vi "MCLB Populate.vi"(6 "Item Names[][]":string[][](array[string]), 8 "error in (no error)":errorcluster, 9 "Column Header Strings[]":string[](array[string]), 10 "Row Header Strings[]":string[](array[string]), 11 "View in":refnum<class "MCListbox View.lvclass">) -> (0 "error out":errorcluster, 3 "View out":refnum<class "MCListbox View.lvclass">)   [LabVIEW 2013, in "SET Project Editor.lvlib" / "MCListbox View.lvclass"]
uses:
  MCListbox View.lvclass
  MCListbox View.lvclass/MCListbox View.ctl
  SET Project Editor.lvlib
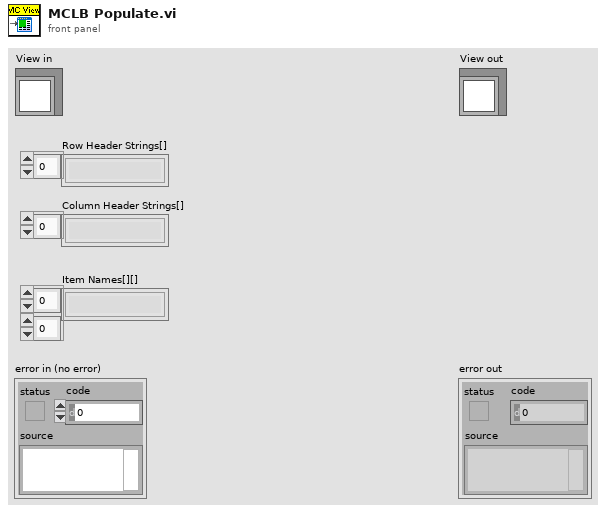
[diagram p1: front panel]
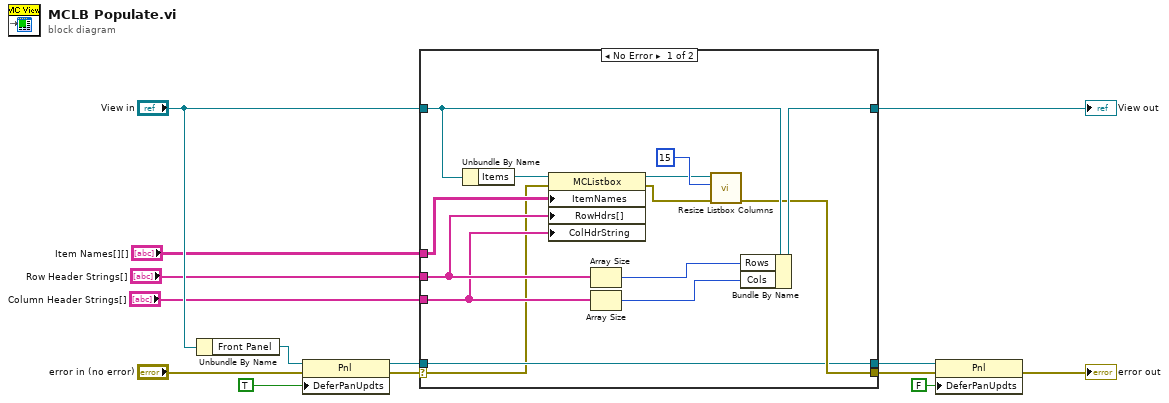
[diagram p0: block diagram]
diagram:
  n1 = Unbundle By Name("View in") -> ("Front Panel"=w12:refnum<vi>)
  n2 = property class="Pnl"(reference=w12, error in="error in (no error)", "DeferPanUpdts"=TRUE ("Defer Panel Updates")) -> (reference out=w8:refnum<vi>, error out=w9:errorcluster)
  n3 = case shown="No Error" w9 {
    selector: w9 -> [w15 w31]
    tunnel: [w22 w31] -> w2
    tunnel: [w26 w30] -> w14
    tunnel: "View in" -> [w27 w30]
    tunnel: w8 -> [w19 w29]
    tunnel: [w19 w29] -> w7
    tunnel: "Item Names[][]" -> [w18 _]
    tunnel: "Row Header Strings[]" -> [w17 _]
    tunnel: "Column Header Strings[]" -> [w16 _]
    frame No Error {
      n4 = Unbundle By Name(w27) -> ("Items"=w28:refnum<vi>)
      n5 = property class="MCListbox"(reference=w28, error in=w15, "ItemNames"=w18, "RowHdrs[]"=w17, "ColHdrString"=w16) -> (reference out=w24:refnum<vi>, error out=w23:errorcluster)
      n6 = Array Size(array=w17) -> (size(s)=w21:i32)
      n7 = Array Size(array=w16) -> (size(s)=w20:i32)
      n8 = call "Resize Listbox Columns.vi"("error in (no error)"=w23, "Padding (5px)"=i16 15, "Listbox Control ref in"=w24) -> ("error out"=w22:errorcluster)  [unwired: 7 in, 1 out]
      n9 = Bundle By Name(cluster=w27, "Rows"=w21, "Cols"=w20) -> (w26:refnum<class "MCListbox View.lvclass">)
    }
    frame Error {
    }
  }
  "View out" <- w14
  n10 = property class="Pnl"(reference=w7, error in=w2, "DeferPanUpdts"=FALSE ("Defer Panel Updates")) -> (error out=→"error out":errorcluster)  [unwired: 1 out]
